vi "Sort Aliases by Names & Decreasing Length.vi"(10 "Definitions Array":string[](array[string]), 11 "Aliases Array":string[](array[string])) -> (2 "Co-sorted Definitions Array":string[](array[string]), 3 "Sorted Aliases Array":string[](array[string]))   [LabVIEW 2021, in "Formula.lvlib"]
uses:
  <userlib>/_OpenG.lib/array/array.llb/Sort 1D Array (String)__ogtk.vi
  <userlib>/_OpenG.lib/array/array.llb/Reorder 1D Array2 (String)__ogtk.vi
  <userlib>/_OpenG.lib/array/array.llb/Sort 1D Array (I32)__ogtk.vi
  Formula.lvlib
  <userlib>/_OpenG.lib/array/array.llb/openg_array.lvlib
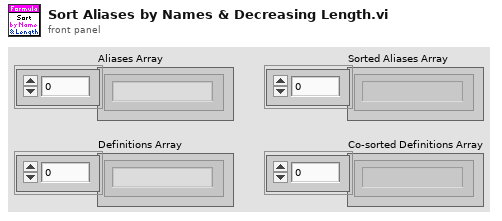
[diagram p1: front panel]
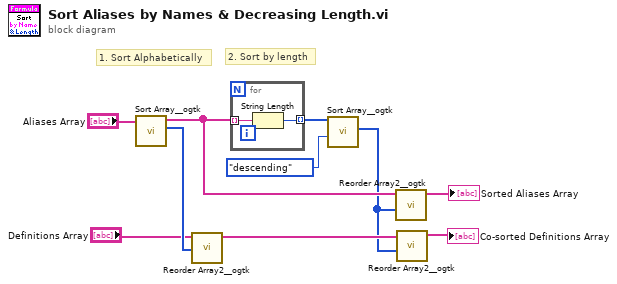
[diagram p0: block diagram]
diagram:
  # "2. Sort by length"
  # "1. Sort Alphabetically"
  n1 = call-poly <userlib>:"Sort Array__ogtk.vi"("Array in"="Aliases Array") -> ("Sorted Pointers"=w9:i32[], "Sorted Array out"=w5:string[])  [unwired: 9 in]
  n2 = call-poly <userlib>:"Reorder Array2__ogtk.vi"("indices"=w9, "array"="Definitions Array") -> ("reordered array"=w4:string[])  [unwired: 9 in]
  n3 = for {
    tunnel: w5 -> [w12] mode=indexing
    tunnel: [w11] -> w7 mode=indexing
    n4 = String Length(string=w12) -> (length=w11:i32)
  }
  n5 = call-poly <userlib>:"Sort Array__ogtk.vi"("Order"=enum16{"ascending", "descending"}."descending", "Array in"=w7) -> ("Sorted Pointers"=w3:i32[])  [unwired: 8 in, 1 out]
  n6 = call-poly <userlib>:"Reorder Array2__ogtk.vi"("indices"=w3, "array"=w5) -> ("reordered array"=→"Sorted Aliases Array":string[])  [unwired: 9 in]
  n7 = call-poly <userlib>:"Reorder Array2__ogtk.vi"("indices"=w3, "array"=w4) -> ("reordered array"=→"Co-sorted Definitions Array":string[])  [unwired: 9 in]
